vi "Display Function Value.vi"(10 "Display Function":T1) -> (2 "DisplayFunc":u8 format="%.0x")   [LabVIEW 2023, in "CTI-Visa-DeviceLib.lvlib" / "LCD-I2C.lvclass"]
uses:
  LCD-I2C.lvclass
  Display Function.ctl
  Bus Mode.ctl
  Lines.ctl
  Glyph Size.ctl
  LCD-I2C.lvclass/LCD-I2C.ctl
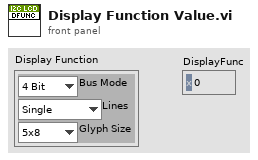
[diagram p1: front panel]
types:
  T1 = typedef "CTI-Visa-DeviceLib.lvlib/LCD-I2C.lvclass/Display Function.ctl" = cluster{"Bus Mode":T2, "Lines":T3, "Glyph Size":T4}
  T2 = typedef "CTI-Visa-DeviceLib.lvlib/LCD-I2C.lvclass/Bus Mode.ctl" = enum8{"4 Bit", "8 Bit"}
  T3 = typedef "CTI-Visa-DeviceLib.lvlib/LCD-I2C.lvclass/Lines.ctl" = enum8{"Single", "Multiline"}
  T4 = typedef "CTI-Visa-DeviceLib.lvlib/LCD-I2C.lvclass/Glyph Size.ctl" = enum8{"5x8", "5x10"}
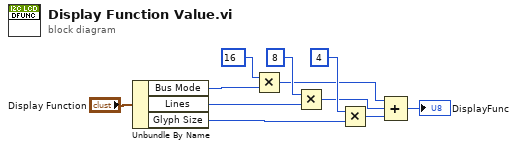
[diagram p0: block diagram]
diagram:
  n1 = Unbundle By Name("Display Function") -> ("Bus Mode"=w9:T2, "Lines"=w7:T3, "Glyph Size"=w5:T4)
  n2 = Multiply(x=u8 16, y=w9) -> (x*y=w1:u8)
  n3 = Multiply(x=u8 8, y=w7) -> (x*y=w2:u8)
  n4 = Multiply(x=u8 4, y=w5) -> (x*y=w3:u8)
  n5 = Compound Arithmetic op=ADD(w1, w2, w3) -> (→"DisplayFunc":u8)
